vi "Process_donotrun.vi"(8 "error in (no error)":errorcluster, 11 "RemoteControl.ZMQ":refnum<class "RemoteControl.ZMQ.lvclass">) -> (0 "error out":errorcluster, 3 "RemoteControl.ZMQ out":refnum<class "RemoteControl.ZMQ.lvclass">)   [LabVIEW 2019, in "RemoteControl.ZMQ.lvclass"]
doc: "---------------------------------------------------------------\nJKI State Machine Objects™\nhttp://jki.net/state-machine-objects/\nCopyright (C) 2005-2015, JKI <info@jki.net>\nALL RIGHTS RESERVED"
uses:
  RemoteControl.ZMQ.lvclass
  <vilib>/JKI/JKI SMO/SMO/SMO.lvclass
  8787fd3b-6c90-4f4d-93f1-f8fb4481aecc.vi
  <userlib>/LevyLab/RemoteControl/RemoteControl.lvclass
  <userlib>/LevyLab/RemoteControl/Typedefs/Message--Cluster.ctl
  <vilib>/JKI/JKI SMO/SMO/Typedefs/Reserve State--Enum.ctl
  <vilib>/JKI/JKI SMO/SMO/Typedefs/SMOState --Enum.ctl
  <vilib>/JKI/JKI SMO/SMO/Typedefs/Public Events.ctl
  <vilib>/addons/zeromq/zmq_context.lvclass
  <vilib>/addons/zeromq/zmq_socket.lvclass
  <vilib>/addons/zeromq/socket_type.ctl
  <vilib>/addons/zeromq/zeromq.lvlib
  C:/Program Files (x86)/National Instruments/LabVIEW 2019/vi.lib/JKI/JKI SMO/SMO/SMO.lvclass
  C:/Program Files (x86)/National Instruments/LabVIEW 2019/user.lib/LevyLab/RemoteControl/RemoteControl.lvclass
panel:
  in  "endpoint":string="tcp://127.0.0.1:5555"
  out "loop":i32
  in  "stop?":bool
  in  "delay response":bool
  in  "timeout (ms) [500]":i32=500
  out "Message In":string
  in  "stop":bool
  out "Message Out":string
  out "State History":string
  # "remote control"
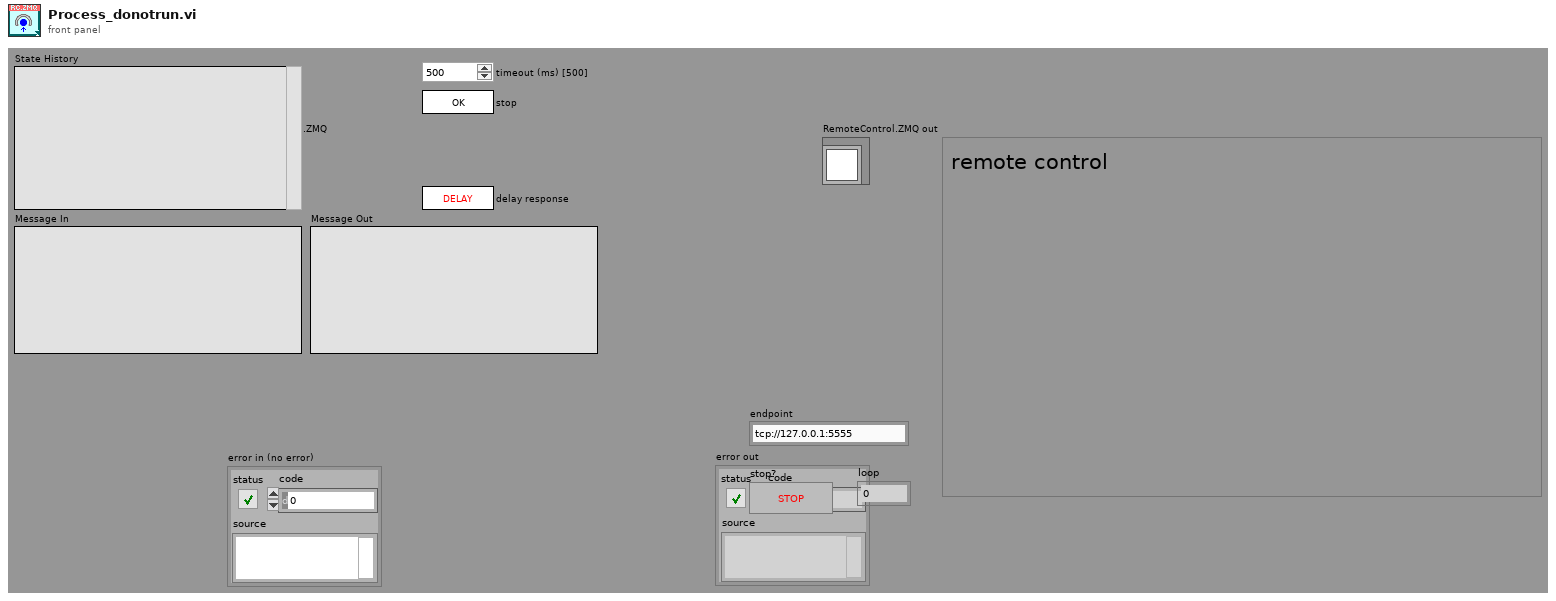
[diagram p1: front panel]
types:
  T1 = enum32{"invalid app kind", "Development System", "Run Time System", "Student Edition", "Embedded LabVIEW", "Evaluation", "Custom"}
  T2 = enum32{"Invalid", "Standard", "Closed", "Hidden", "Minimized", "Maximized"}
  T3 = enum32{"Bad", "Idle", "Run top level", "Running"}
  T4 = typedef "RemoteControl.lvclass/Message--Cluster.ctl" = cluster{"Command":string, "Data":variant, "ID":string}
  T5 = typedef "zeromq.lvlib/socket_type.ctl" = enum8{"ZMQ_PAIR", "ZMQ_PUB", "ZMQ_SUB", "ZMQ_REQ", "ZMQ_REP", "ZMQ_DEALER", "ZMQ_ROUTER", "ZMQ_PULL", "ZMQ_PUSH", "ZMQ_XPUB", "ZMQ_XSUB", "ZMQ_STREAM", "ZMQ_SERVER", "ZMQ_CLIENT", "ZMQ_RADIO", "ZMQ_DISH", "ZMQ_GATHER", "ZMQ_SCATTER", "ZMQ_DGRAM"}
  T6 = cluster{"Core":cluster{"Current VI Reference":refnum<vi>, "Close Panel on Exit?":bool, "Last Error":cluster{"error":errorcluster, "previous state":string, "remaining states":string}, "Shutdown?":bool}, "SelfRef":refnum<class "RemoteControl.ZMQ.lvclass">, "Message (in)":T4, "Message (out)":T4, "state":enum16{"waiting", "processing"}, "to":i32}
  T7 = cluster{"Current VI Reference":refnum<vi>, "Close Panel on Exit?":bool, "Last Error":cluster{"error":errorcluster, "previous state":string, "remaining states":string}, "Shutdown?":bool}
  T8 = typedef "SMO.lvclass/Public Events.ctl" = cluster{"Error":refnum<user-event>, "State":refnum<user-event>, "Reserve State":refnum<user-event>}
  T9 = typedef "SMO.lvclass/Protected Events.ctl" = cluster{"StopProcesses":refnum<user-event>, "AbortProcesses":refnum<user-event>, "Config Changed":refnum<user-event>, "Dependency":refnum<user-event>}
  T10 = typedef "RemoteControl.lvclass/PrivateEvents--Cluster.ctl" = cluster{"Configure":refnum<user-event>, "SendMessageToProcess":refnum<user-event>}
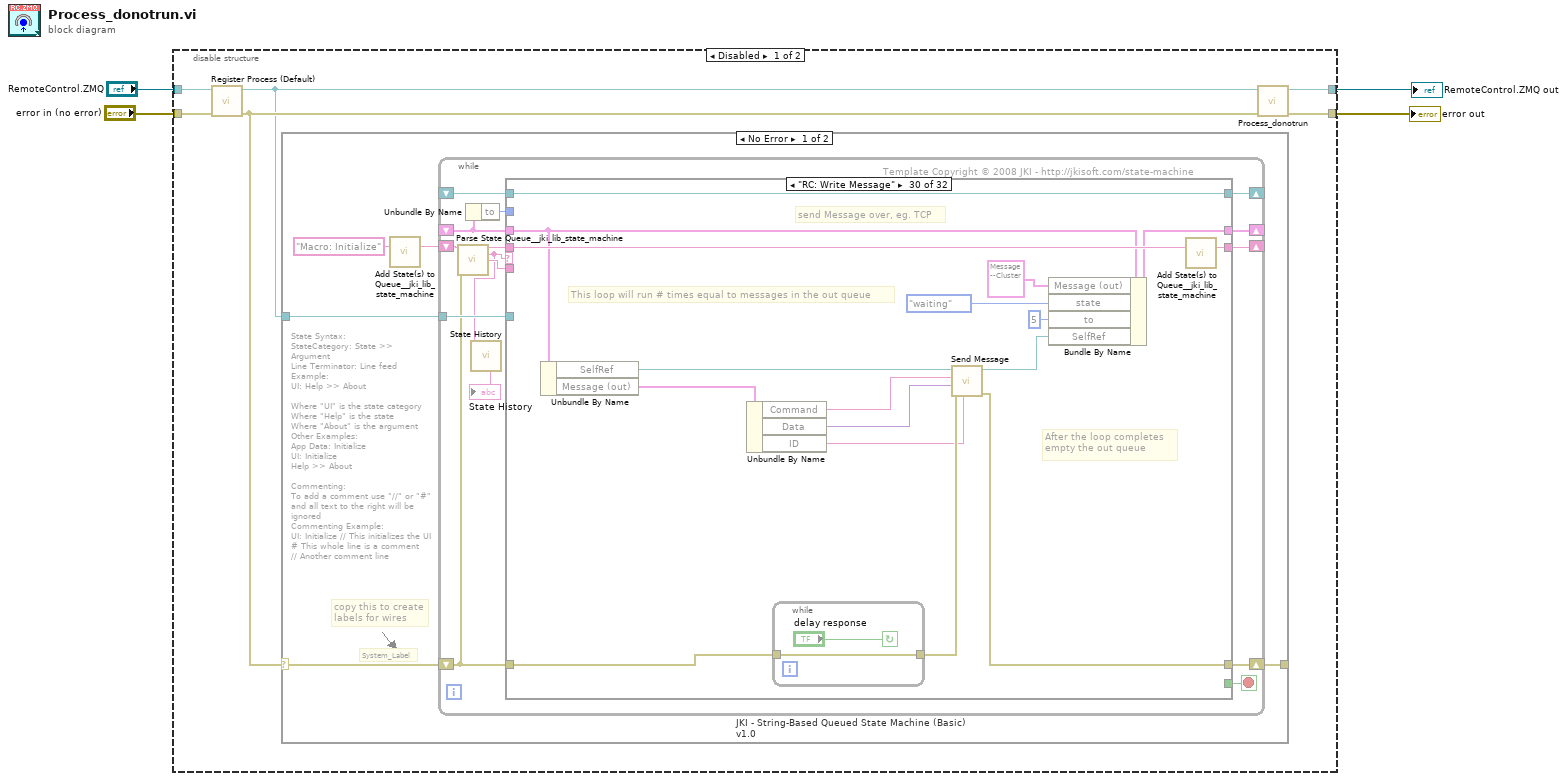
[diagram p0: block diagram]
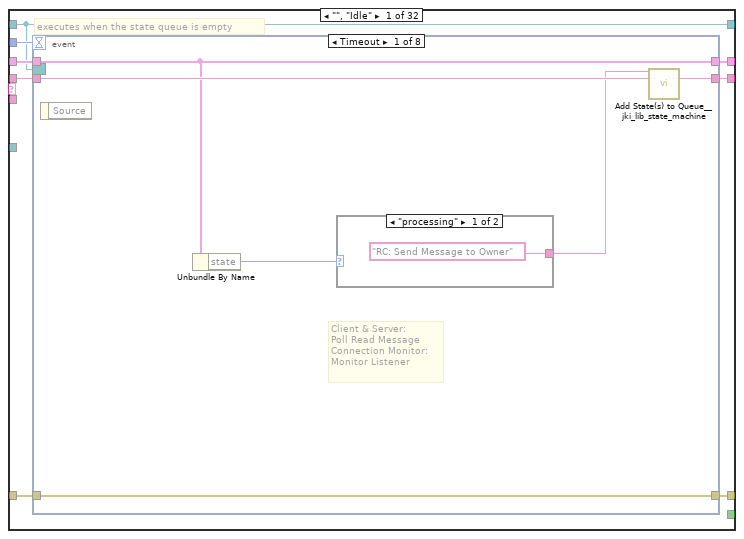
[diagram p2: hidden frame]
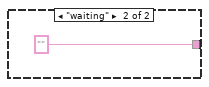
[diagram p3: hidden frame]
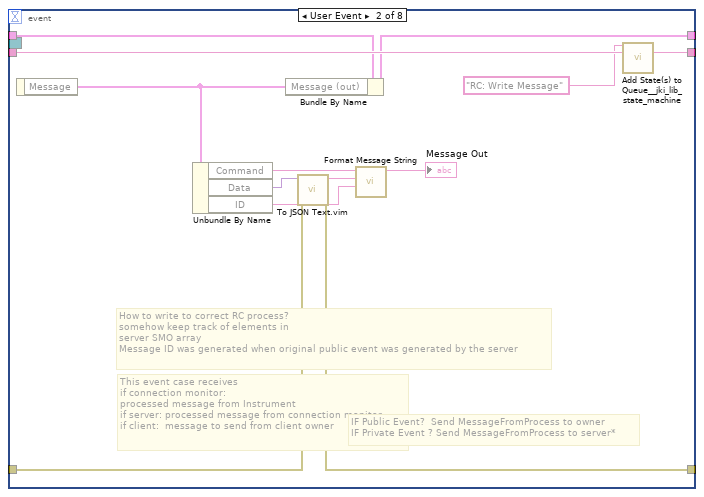
[diagram p4: hidden frame]
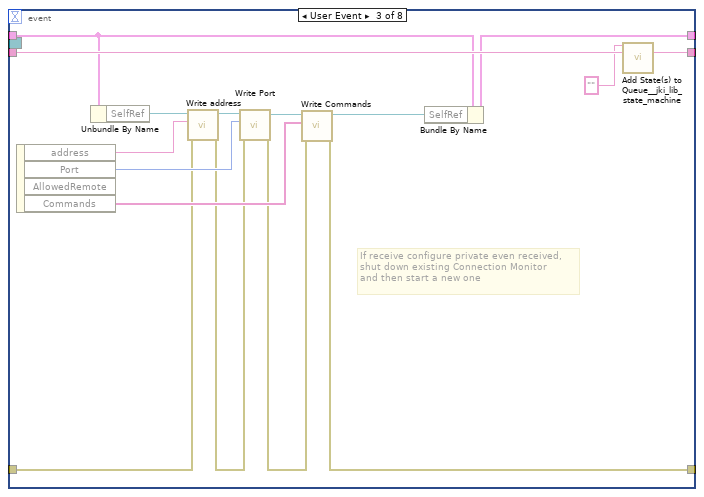
[diagram p5: hidden frame]
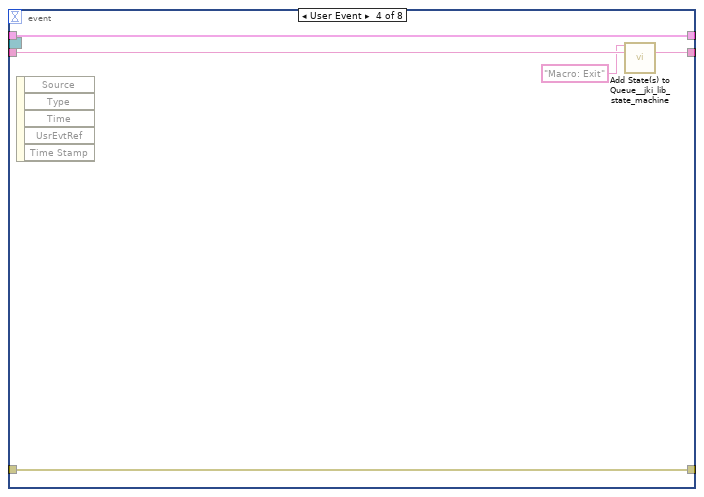
[diagram p6: hidden frame]
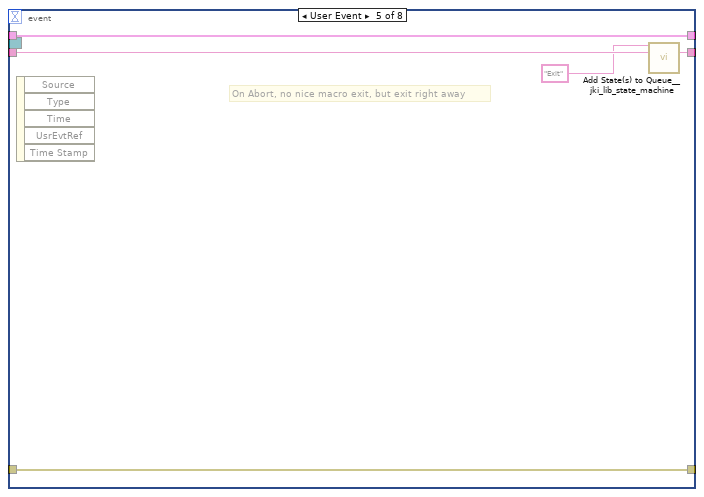
[diagram p7: hidden frame]
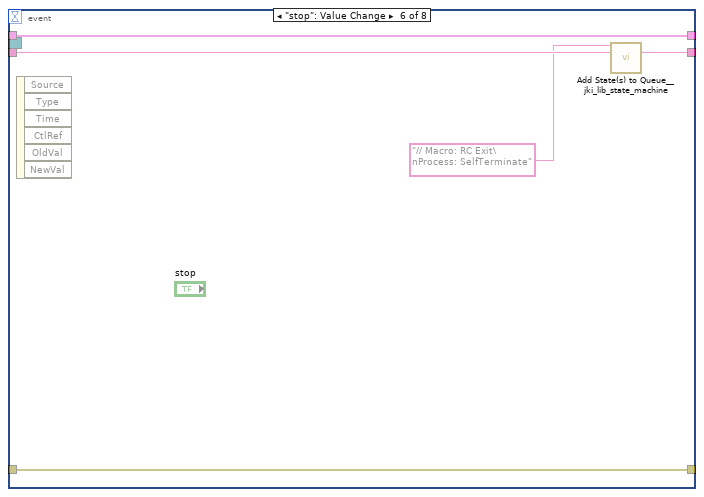
[diagram p8: hidden frame]
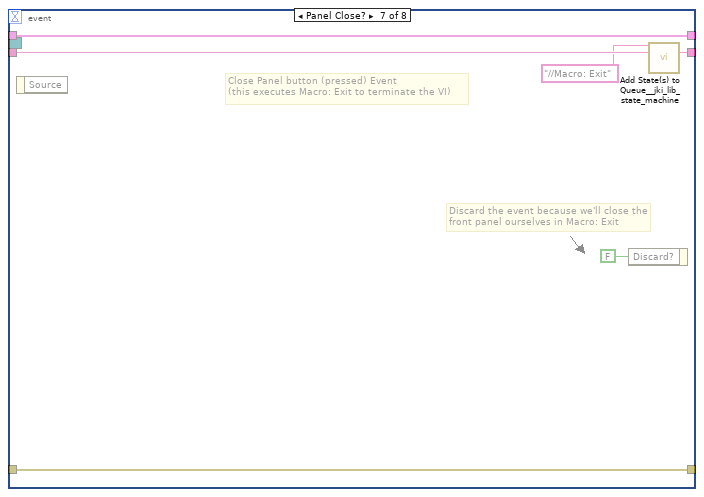
[diagram p9: hidden frame]
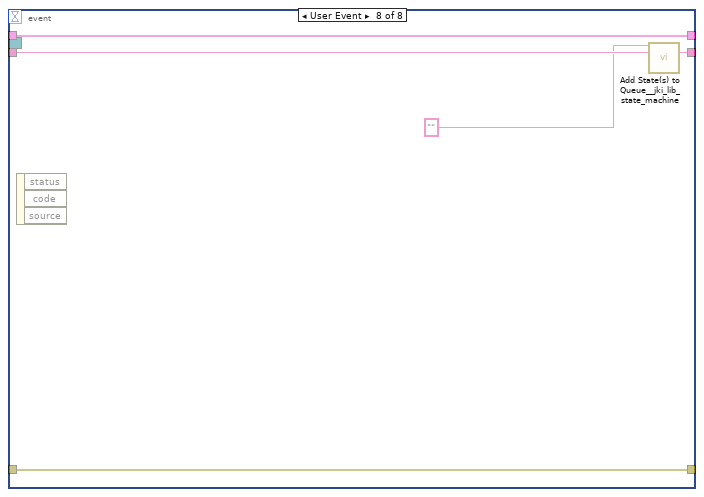
[diagram p10: hidden frame]
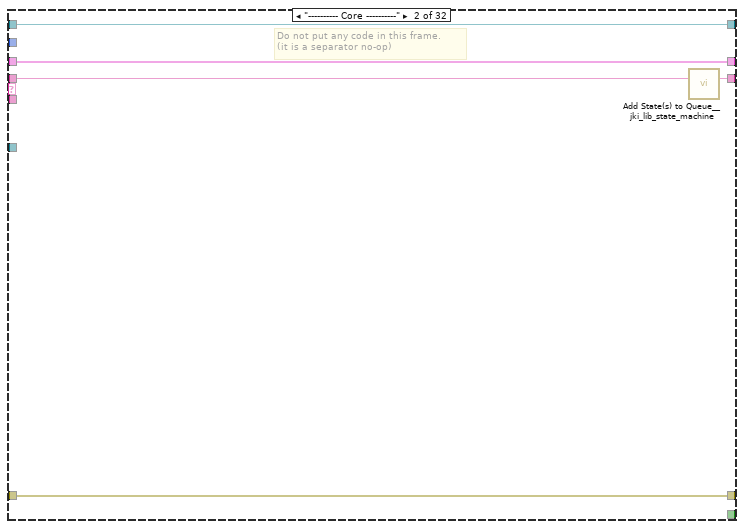
[diagram p11: hidden frame]
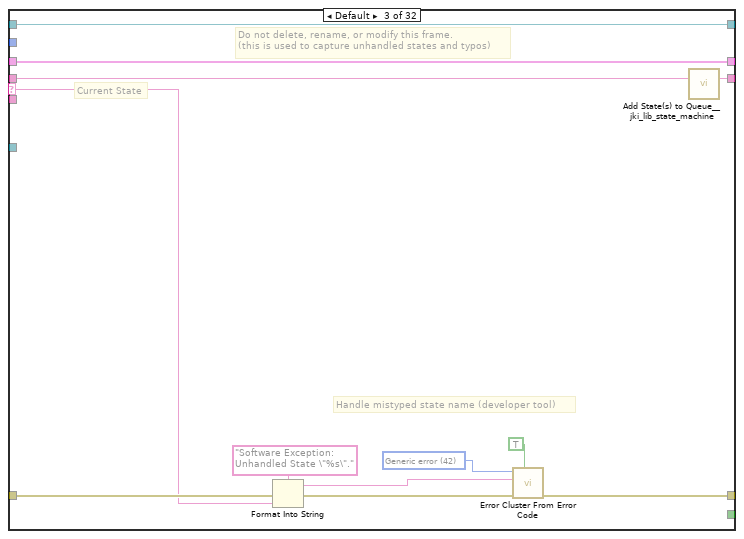
[diagram p12: hidden frame]
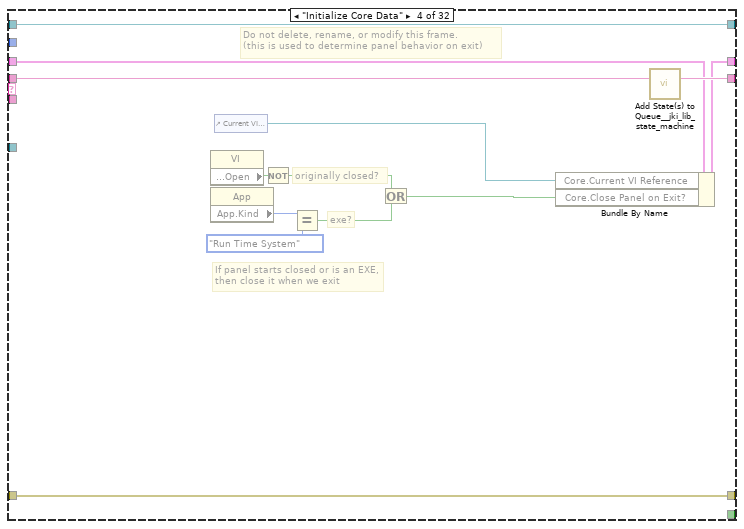
[diagram p13: hidden frame]
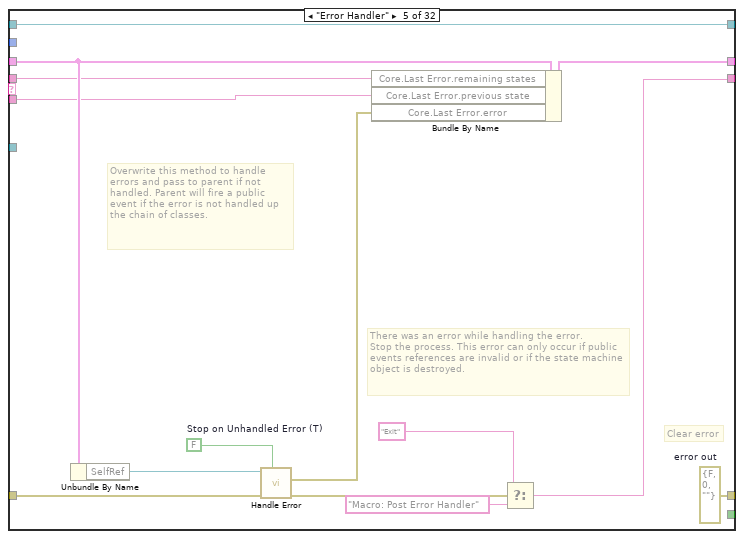
[diagram p14: hidden frame]
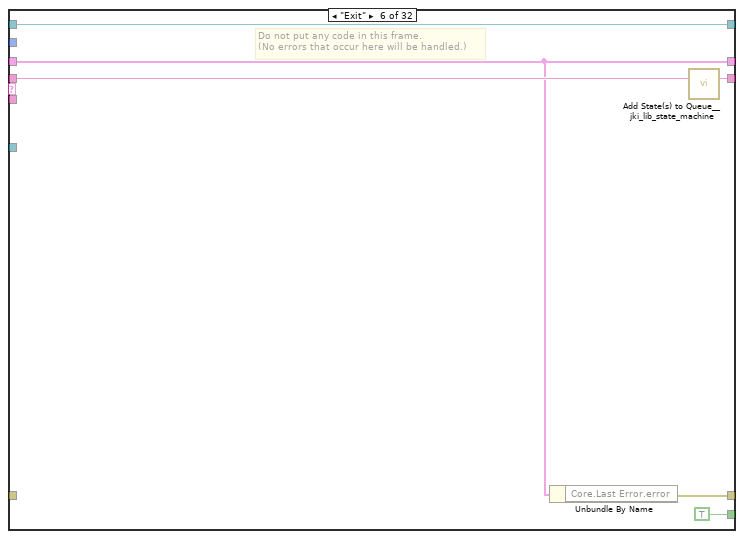
[diagram p15: hidden frame]
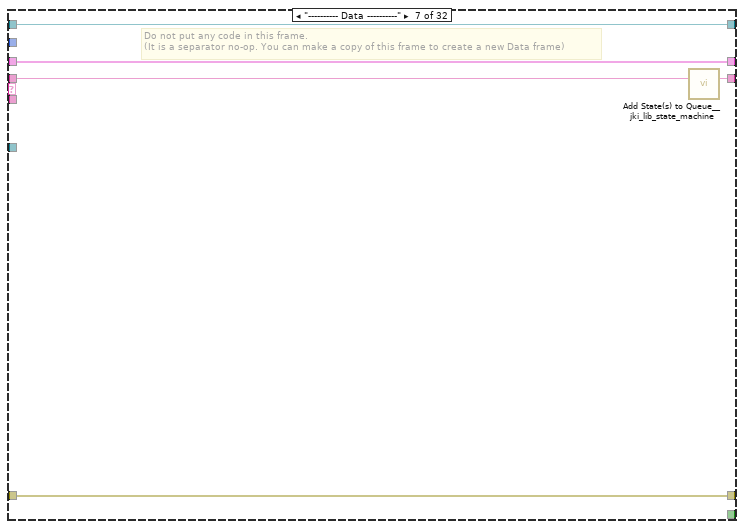
[diagram p16: hidden frame]
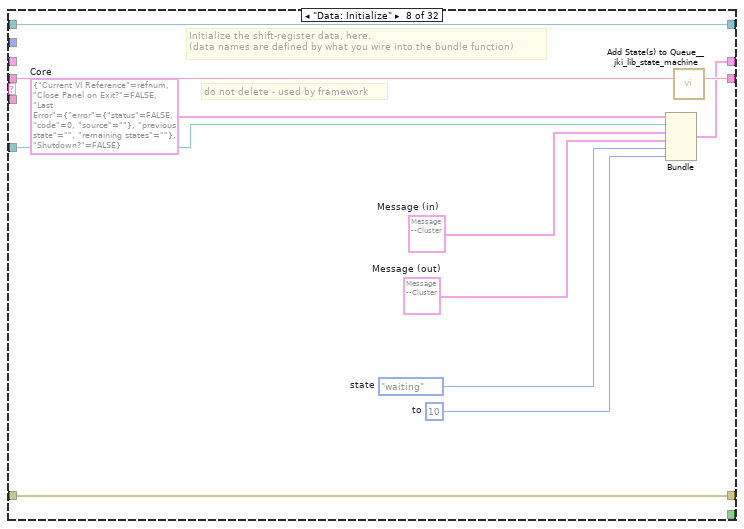
[diagram p17: hidden frame]
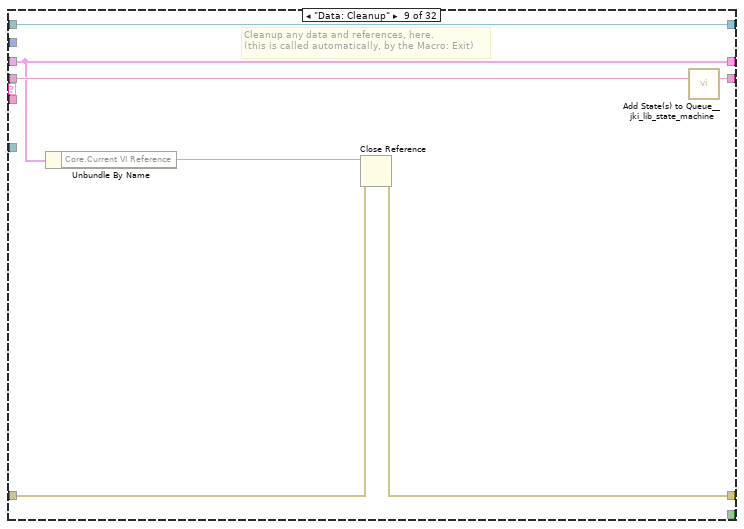
[diagram p18: hidden frame]
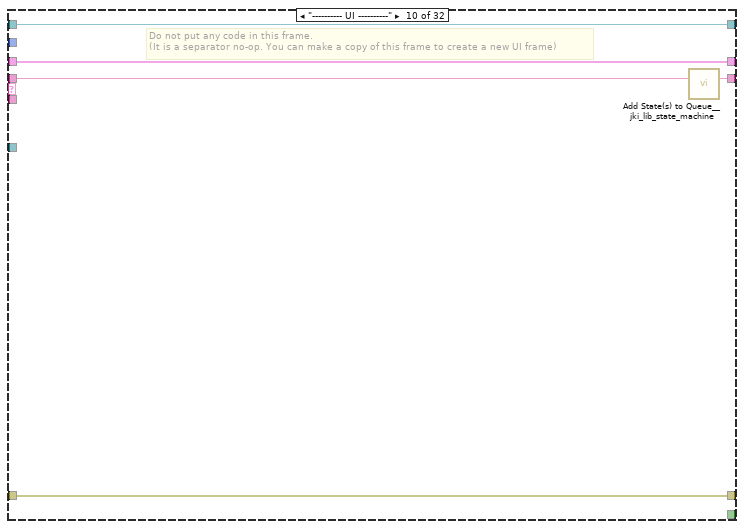
[diagram p19: hidden frame]
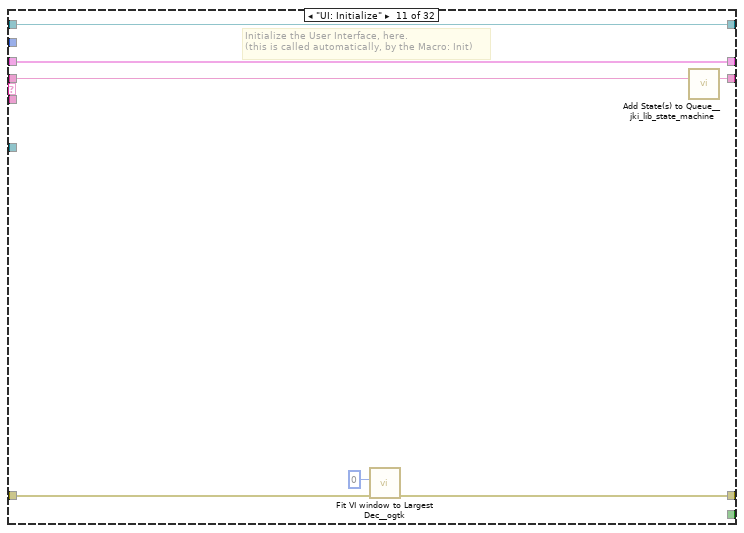
[diagram p20: hidden frame]
diagram:
  n1 = disable-structure shown="Disabled" {
    disable-tunnel: "RemoteControl.ZMQ" -> [w10 w465]
    disable-tunnel: "error in (no error)" -> [w9 w464]
    disable-tunnel: [w6 w465] -> w2
    disable-tunnel: [w5 w464] -> w1
    frame Disabled {
      n2 = call <vilib>:"Register Process (Default).vi"("error in (no error)"=w9, "SMO"=w10) -> ("error out"=w8:errorcluster, "SelfRef"=w7:refnum<class "RemoteControl.ZMQ.lvclass">)  [unwired: 8 in]
      n3 = case shown="No Error" w8 {
        selector: w8 -> [w12 w463]
        tunnel: w7 -> [w13 _]
        tunnel: [w11 w463] -> _
        frame No Error {
          # "State Syntax:\nStateCategory: State >> Argument\nLine Terminator: Line feed\nExample:\nUI: Help >> About\n\nWhere \"UI\" is the state category\nWhere \"Help\" is the state\nWhere \"About\" is the argument\nOther Examples:\nApp Data: Initialize\nUI: Initialize\nHelp >> About\n\nCommenting:\nTo add a comment use \"//\" or \"#\" and all text to the right will be ignored\nCommenting Example:\nUI: Initialize // This initializes the UI\n# This whole line is a comment\n// Another comment line"
          # "copy this to create labels for wires"
          # "System_Label"
          n4 = call <vilib>:"Add State(s) to Queue__jki_lib_state_machine.vi"("State(s) in (\"\")"="Macro: Initialize") -> ("States Out"=w15:string)  [unwired: 14 in]
          n5 = while "JKI - String-Based Queued State Machine (Basic) v1.0" {
            shift-right: [w25] -> _
            shift-left: _ -> [w18]
            shift-right: [w27] -> w11
            shift-left: w12 -> [w21]
            shift-right: [w19] -> _
            shift-left: w15 -> [w28]
            tunnel: w13 -> [w24]
            shift-right: [w23] -> _
            shift-left: _ -> [w22]
            stop <- w26 stop-if-true
            # "Template Copyright © 2008 JKI - http://jkisoft.com/state-machine"
            n6 = call <vilib>:"Parse State Queue__jki_lib_state_machine.vi"("State Queue"=w28, "Error In (no error)"=w21) -> ("Remaining States"=w30:string, "Current State"=w20:string, "Arguments"=w29:string)  [unwired: 11 in]
            n7 = Unbundle By Name(w18) -> ("to"=w17:i32)
            n8 = call <userlib>:"State History.vi"("Current State"=w20) -> ("History"=→"State History":string)  [unwired: 10 in]
            n9 = case shown="\"RC: Write Message\"" w20 {
              selector: w20 -> [_ _ w108 _ _ _ _ _ _ _ _ _ _ _ _ _ _ _ _ _ _ _ _ _ _ _ _ _ _ _ _ _]
              tunnel: w30 -> [w38 w106 w112 w131 w135 w151 w156 w167 w174 w179 w186 w193 w209 w239 w244 w266 w272 w278 w292 w316 w321 w332 w341 w346 w360 w366 w371 w379 w402 w436 w447 w462]
              tunnel: w29 -> [_ _ _ _ w134 _ _ _ _ _ _ w187 w204 _ _ _ _ _ _ _ _ _ _ _ _ _ _ _ _ _ _ _]
              tunnel: [w35 w104 w114 w128 w144 w146 w154 w160 w171 w177 w181 w188 w202 w235 w242 w264 w269 w276 w290 w314 w319 w324 w334 w344 w354 w362 w367 w374 w395 w431 w439 w459] -> w27
              tunnel: [w37 w105 w111 w130 w137 w150 w155 w166 w173 w178 w185 w192 w208 w238 w243 w265 w271 w277 w291 w315 w320 w331 w340 w345 w359 w365 w370 w378 w401 w435 w446 w461] -> w19
              tunnel: [_ _ _ _ _ TRUE _ _ _ _ _ _ _ _ _ _ _ _ _ _ _ _ _ _ _ _ _ _ _ _ _ _] -> w26
              tunnel: [w33 w103 w110 w129 w142 w147 w153 w163 w170 w176 w183 w191 w206 w236 w241 w246 w268 w273 w288 w300 w318 w329 w338 w343 w358 w364 w369 w375 w399 w429 w442 w457] -> w25
              tunnel: w17 -> [w32 _ _ _ _ _ _ _ _ _ _ _ _ _ _ _ _ _ _ _ _ _ _ _ _ _ _ _ _ _ _ _]
              tunnel: w24 -> [_ _ _ _ _ _ _ w157 _ _ _ _ _ _ _ _ _ _ _ _ _ _ _ _ _ _ _ _ _ _ _ _]
              tunnel: [w31 w102 w107 w119 w145 w148 w152 w165 w169 w175 w184 w190 w203 w237 w240 w263 w270 w275 w289 w310 w317 w330 w339 w342 w357 w363 w368 w377 w400 w434 w445 w460] -> w23
              tunnel: w22 -> [w31 w102 w107 w119 w145 w148 w152 w165 w169 w175 w184 w190 w203 w237 w240 w263 w270 w275 w289 w310 w317 w330 w339 w342 _ w363 w368 w377 w400 w434 w445 w460]
              tunnel: w21 -> [w34 w104 w113 w128 w140 _ w154 w160 w172 w177 w180 w189 w207 w235 w242 w264 w269 w276 w290 w314 w319 w325 w335 w344 w355 w362 w367 w373 w385 w432 w440 w449]
              tunnel: w18 -> [w36 w103 w110 w122 w143 w147 w153 _ w170 w176 w183 w191 w206 w236 w241 w246 w268 w273 w286 w299 w318 w329 w333 w343 w358 w364 w369 w375 w387 w430 w443 w456]
              frame "", "Idle" {
                # "executes when the state queue is empty"
                n10 = event shown="[0] Timeout" {
                  selector: w31 -> [_ _ _ _ _ _ _ _]
                  dyn-events: _ -> [_ _ _ _ _ _ _ _]
                  timeout: w32 -> [_ _ _ _ _ _ _ _]
                  tunnel: w38 -> [w44 w59 w75 w80 w85 w89 w96 w101]
                  tunnel: [w43 w58 w74 w79 w84 w90 w95 w100] -> w37
                  tunnel: w36 -> [w40 w55 w66 w77 w82 w88 w93 w98]
                  tunnel: [w42 w48 w60 w78 w83 w86 w94 w99] -> w35
                  tunnel: w34 -> [w42 w47 w62 w78 w83 w86 w94 w99]
                  tunnel: [w40 w57 w73 w77 w82 w88 w93 w98] -> w33
                  event Timeout {
                    # "Client & Server:\nPoll Read Message\nConnection Monitor:\nMonitor Listener"
                    n11 = event-data() -> ()  [unwired: 1 in, 1 out]
                    n12 = Unbundle By Name(w40) -> ("state"=w39:enum16{"waiting", "processing"})
                    n13 = case shown="\"processing\"" w39 {
                      tunnel: ["RC: Send Message to Owner" ("State(s) in Front (\"\")") "" ("State(s) in Front (\"\")")] -> w41
                      frame "processing" {
                      }
                      frame "waiting" {
                      }
                    }
                    n14 = call <vilib>:"Add State(s) to Queue__jki_lib_state_machine.vi"("State(s) in Front (\"\")"=w41, "State(s) in (\"\")"=w44) -> ("States Out"=w43:string)  [unwired: 13 in]
                  }
                  event User Event {
                    # "IF Public Event?  Send MessageFromProcess to owner\nIF Private Event ? Send MessageFromProcess to server*"
                    # "How to write to correct RC process?\nsomehow keep track of elements in\nserver SMO array\nMessage ID was generated when original public event was generated by the server"
                    # "This event case receives\nif connection monitor:\nprocessed message from Instrument\nif server: processed message from connection monitor\nif client:  message to send from client owner"
                    n15 = event-data() -> ("Message"=w49:T4)  [unwired: 1 in]
                    n16 = Unbundle By Name(w49) -> ("Command"=w52:string, "Data"=w51:variant, "ID"=w50:string)
                    n17 = Bundle By Name(cluster=w55, "Message (out)"=w49) -> (w57:T6)
                    n18 = call "To JSON Text.vim"("error in (no error)"=w47, "Anything"=w51) -> ("error out"=w48:errorcluster, "<JSON>"=w53:string)  [unwired: 8 in]
                    n19 = call <userlib>:"Format Message String.vi"("ID"=w50, "Data"=w53, "Command"=w52) -> ("Message"=→"Message Out":string)  [unwired: 8 in]
                    n20 = call <vilib>:"Add State(s) to Queue__jki_lib_state_machine.vi"("State(s) in Front (\"\")"="RC: Write Message" ("State(s) in Front (\"\")"), "State(s) in (\"\")"=w59) -> ("States Out"=w58:string)  [unwired: 13 in]
                  }
                  event User Event {
                    # "If receive configure private even received,\nshut down existing Connection Monitor \nand then start a new one"
                    n21 = event-data() -> ("address"=w64:string, "Port"=w71:u16, "Commands"=w70:string[])  [unwired: 1 in, 1 out]
                    n22 = Unbundle By Name(w66) -> ("SelfRef"=w65:refnum<class "RemoteControl.ZMQ.lvclass">)
                    n23 = call-dynamic "Write address.vi"("error in (no error)"=w62, "address"=w64, "RemoteControl in"=w65) -> ("error out"=w63:errorcluster, "RemoteControl out"=w68:refnum<class "RemoteControl.ZMQ.lvclass">)  [unwired: 7 in]
                    n24 = call-dynamic "Write Port.vi"("error in (no error)"=w63, "Port"=w71, "RemoteControl in"=w68) -> ("error out"=w61:errorcluster, "RemoteControl out"=w69:refnum<class "RemoteControl.ZMQ.lvclass">)  [unwired: 7 in]
                    n25 = call-dynamic "Write Commands.vi"("error in (no error)"=w61, "Commands"=w70, "RemoteControl in"=w69) -> ("error out"=w60:errorcluster, "RemoteControl out"=w67:refnum<class "RemoteControl.ZMQ.lvclass">)  [unwired: 7 in]
                    n26 = Bundle By Name(cluster=w66, "SelfRef"=w67) -> (w73:T6)
                    n27 = call <vilib>:"Add State(s) to Queue__jki_lib_state_machine.vi"("State(s) in Front (\"\")"="" ("State(s) in Front (\"\")"), "State(s) in (\"\")"=w75) -> ("States Out"=w74:string)  [unwired: 13 in]
                  }
                  event User Event {
                    n28 = event-data() -> ()  [unwired: 1 in, 5 out]
                    n29 = call <vilib>:"Add State(s) to Queue__jki_lib_state_machine.vi"("State(s) in Front (\"\")"="Macro: Exit", "State(s) in (\"\")"=w80) -> ("States Out"=w79:string)  [unwired: 13 in]
                  }
                  event User Event {
                    # "On Abort, no nice macro exit, but exit right away"
                    n30 = event-data() -> ()  [unwired: 1 in, 5 out]
                    n31 = call <vilib>:"Add State(s) to Queue__jki_lib_state_machine.vi"("State(s) in Front (\"\")"="Exit", "State(s) in (\"\")"=w85) -> ("States Out"=w84:string)  [unwired: 13 in]
                  }
                  event "stop": Value Change {
                    n32 = event-data() -> ()  [unwired: 1 in, 6 out]
                    n33 = call <vilib>:"Add State(s) to Queue__jki_lib_state_machine.vi"("State(s) in Front (\"\")"="// Macro: RC Exit\nProcess: SelfTerminate" ("State(s) in Front (\"\")"), "State(s) in (\"\")"=w89) -> ("States Out"=w90:string)  [unwired: 13 in]
                  }
                  event Panel Close? {
                    # "Discard the event because we'll close the front panel ourselves in Macro: Exit"
                    # "Close Panel button (pressed) Event\n(this executes Macro: Exit to terminate the VI)"
                    n34 = event-data() -> ()  [unwired: 1 in, 1 out]
                    n35 = event-data("Discard?"=FALSE) -> ()  [unwired: 1 in, 1 out]
                    n36 = call <vilib>:"Add State(s) to Queue__jki_lib_state_machine.vi"("State(s) in Front (\"\")"="//Macro: Exit", "State(s) in (\"\")"=w96) -> ("States Out"=w95:string)  [unwired: 13 in]
                  }
                  event User Event {
                    n37 = event-data() -> ()  [unwired: 1 in, 3 out]
                    n38 = call <vilib>:"Add State(s) to Queue__jki_lib_state_machine.vi"("State(s) in Front (\"\")"="", "State(s) in (\"\")"=w101) -> ("States Out"=w100:string)  [unwired: 13 in]
                  }
                }
              }
              frame "---------- Core ----------" {
                # "Do not put any code in this frame.\n(it is a separator no-op)"
                n39 = call <vilib>:"Add State(s) to Queue__jki_lib_state_machine.vi"("State(s) in (\"\")"=w106) -> ("States Out"=w105:string)  [unwired: 14 in]
              }
              frame Default {
                w117 = 42 items=["No error", "Argument error", "Memory is full", "Out of zone", "End of file", "File already open", "Generic file I/O error", "File not found", "File permission error", "Disk is full", "Duplicate path", "Too many files open", "System feature not enabled", "Resource file not found", "Cannot add resource", "Resource not found", "Image not found", "Image memory error", "Pen does not exist", "Config type invalid", "Config token not found", "Config parse error", "Config memory error", "Bad external code format", "Bad external code offset", "External code not present", "Null window", "Destroy window error", "Null menu", "Print aborted", "Bad print record", "Print driver error", "Windows error during printing", "Memory error during printing", "Print dialog error", "Generic print error", "Invalid device refnum", "Device not found", "Device parameter error", "Device unit error", "Cannot open device", "Device call aborted", "Generic error", "Cancelled by user", "Object ID too low", "Object ID too high", "Object not in heap", "Unknown heap", "Unknown object (invalid DefProc)", "Unknown object (DefProc not in table)", "Message out of range", "Invalid (null) method", "Unknown message", "Manager call not supported", "Bad address", "Network operation in progress", "Network operation timed out", "Connection is busy", "Network attribute not supported", "Network error", "Address in use", "System out of memory", "Connection aborted", "Connection refused", "Not connected", "Already connected", "Connection closed", "Initialization error (interapplication manager)", "Bad occurrence", "Wait on unbound occurrence handler", "Occurrence queue overflow", "Datalog type conflict", "Unused", "Unrecognized type (interapplication manager)", "Memory corrupt", "Failed to make temporary DLL", "Old CIN version", "Drag socket not found", "Failed to load drop-object", "Failed to register OLE object", "Failed to release OLE object", "Format specifier type mismatch", "Unknown format specifier", "Too few format specifiers", "Too many format specifiers", "Scan failed", "Newer CIN version", "Error converting to variant", "Runtime menu error", "Password tampered", "Variant attribute not found", "Incompatible variant data type", "Event data is not available", "Event Store is not present", "Occurrence is not found", "Event Queue is not created", "Event info is not available", "Refnum passed is NULL", "Error retrieving Class GUID", "Error retrieving CoClass GUID", "Error retrieving TypeLib GUID.", "Bad built application magic bytes.", "Specific driver is different from the specific driver associated with the Logical Name.", "There is no session opened to the class driver.", "Max Error", "MAX - Error with config objects", "MAX - Error loading configuration", "MAX - Group not supported"]
                # "Current State"
                # "Do not delete, rename, or modify this frame.\n(this is used to capture unhandled states and typos)"
                # "Handle mistyped state name (developer tool)"
                n40 = Format Into String(format string="Software Exception: Unhandled State \"%s\"." ("message"), error in=w113, w108) -> (resulting string=w116:string, error out=w115:errorcluster)  [unwired: 1 in]
                n41 = call <vilib>:"Error Cluster From Error Code.vi"("show call chain? (False)"=TRUE, "error in (no error)"=w115, "error message (\"\")"=w116, "error code (0)"=w117) -> ("error out"=w114:errorcluster)  [unwired: 5 in]
                n42 = call <vilib>:"Add State(s) to Queue__jki_lib_state_machine.vi"("State(s) in (\"\")"=w112) -> ("States Out"=w111:string)  [unwired: 14 in]
              }
              frame "Initialize Core Data" {
                # "Do not delete, rename, or modify this frame.\n(this is used to determine panel behavior on exit)"
                # "originally closed?"
                # "exe?"
                # "If panel starts closed or is an EXE, then close it when we exit"
                n43 = property class="VI"() -> ("Front Panel.Open"=w127:bool)  [unwired: 2 in, 2 out]
                n44 = property class="App"() -> ("App.Kind"=w126:T1)  [unwired: 2 in, 2 out]
                n45 = control-ref of="Current VI Reference"() -> (w120:refnum<vi>)
                n46 = Not(x=w127) -> (.not. x?=w124:bool)
                n47 = Equal?(x=w126, y=T1."Run Time System" ("Application:Kind")) -> (x = y?=w123:bool)
                n48 = Or(x=w124, y=w123) -> (x .or. y?=w121:bool)
                n49 = Bundle By Name(cluster=w122, "Core.Current VI Reference"=w120, "Core.Close Panel on Exit?"=w121) -> (w129:T6)
                n50 = call <vilib>:"Add State(s) to Queue__jki_lib_state_machine.vi"("State(s) in (\"\")"=w131) -> ("States Out"=w130:string)  [unwired: 14 in]
              }
              frame "Error Handler" {
                w141 = FALSE  # Stop on Unhandled Error (T)
                w144 = errorcluster {"status"=FALSE, "code"=0, "source"=""}  # error out
                # "There was an error while handling the error.\nStop the process. This error can only occur if public events references are invalid or if the state machine object is destroyed."
                # "Clear error"
                # "Overwrite this method to handle errors and pass to parent if not handled. Parent will fire a public event if the error is not handled up the chain of classes."
                n51 = Unbundle By Name(w143) -> ("SelfRef"=w139:refnum<class "RemoteControl.ZMQ.lvclass">)
                n52 = call-dynamic "Handle Error.vi"("Stop on Unhandled Error (T)"=w141, "error in"=w140, "SMO"=w139) -> ("handling error"=w132:errorcluster, "Unhandled error"=w133:errorcluster)  [unwired: 6 in, 1 out]
                n53 = Bundle By Name(cluster=w143, "Core.Last Error.remaining states"=w135, "Core.Last Error.previous state"=w134, "Core.Last Error.error"=w133) -> (w142:T6)
                n54 = Select(t="Exit", s=w132, f="Macro: Post Error Handler") -> (s? t:f=w137:string)
              }
              frame "Exit" {
                # "Do not put any code in this frame.\n(No errors that occur here will be handled.)"
                n55 = Unbundle By Name(w147) -> ("Core.Last Error.error"=w146:errorcluster)
                n56 = call <vilib>:"Add State(s) to Queue__jki_lib_state_machine.vi"("State(s) in (\"\")"=w151) -> ("States Out"=w150:string)  [unwired: 14 in]
              }
              frame "---------- Data ----------" {
                # "Do not put any code in this frame.\n(It is a separator no-op. You can make a copy of this frame to create a new Data frame)"
                n57 = call <vilib>:"Add State(s) to Queue__jki_lib_state_machine.vi"("State(s) in (\"\")"=w156) -> ("States Out"=w155:string)  [unwired: 14 in]
              }
              frame "Data: Initialize" {
                w158 = 10  # to
                w159 = enum16{"waiting", "processing"}."waiting"  # state
                w161 = T4 {"Command"="", "Data"=variant, "ID"=""}  # Message (out)
                w162 = T4 {"Command"="", "Data"=variant, "ID"=""}  # Message (in)
                w164 = T7 {"Current VI Reference"=refnum, "Close Panel on Exit?"=FALSE, "Last Error"={"error"={"status"=FALSE, "code"=0, "source"=""}, "previous state"="", "remaining states"=""}, "Shutdown?"=FALSE}  # Core
                # "do not delete - used by framework"
                # "Initialize the shift-register data, here.\n(data names are defined by what you wire into the bundle function)"
                n58 = Bundle("Core"=w164, "SelfRef"=w157, "Message (in)"=w162, "Message (out)"=w161, "state"=w159, "to"=w158) -> (w163:T6)  [unwired: 1 in]
                n59 = call <vilib>:"Add State(s) to Queue__jki_lib_state_machine.vi"("State(s) in (\"\")"=w167) -> ("States Out"=w166:string)  [unwired: 14 in]
              }
              frame "Data: Cleanup" {
                # "Cleanup any data and references, here.\n(this is called automatically, by the Macro: Exit)"
                n60 = Unbundle By Name(w170) -> ("Core.Current VI Reference"=w168:refnum<vi>)
                n61 = Close Reference(reference=w168, error in (no error)=w172) -> (error out=w171:errorcluster)
                n62 = call <vilib>:"Add State(s) to Queue__jki_lib_state_machine.vi"("State(s) in (\"\")"=w174) -> ("States Out"=w173:string)  [unwired: 14 in]
              }
              frame "---------- UI ----------" {
                # "Do not put any code in this frame.\n(It is a separator no-op. You can make a copy of this frame to create a new UI frame)"
                n63 = call <vilib>:"Add State(s) to Queue__jki_lib_state_machine.vi"("State(s) in (\"\")"=w179) -> ("States Out"=w178:string)  [unwired: 14 in]
              }
              frame "UI: Initialize" {
                # "Initialize the User Interface, here.\n(this is called automatically, by the Macro: Init)"
                n64 = call <userlib>:"Fit VI window to Largest Dec__ogtk.vi"("error in (no error)"=w180, "border spacing (2 px)"=0) -> ("error out"=w181:errorcluster)  [unwired: 4 in, 1 out]
                n65 = call <vilib>:"Add State(s) to Queue__jki_lib_state_machine.vi"("State(s) in (\"\")"=w186) -> ("States Out"=w185:string)  [unwired: 14 in]
              }
              frame "UI: Cursor Set" {
                # "Argument"
                # "Initialize the User Interface, here.\n(this is called automatically, by the Macro: Init)"
                n66 = disable-structure shown="Default" {
                  disable-tunnel: w189 -> [w194 w197]
                  disable-tunnel: [w194 w196] -> w188
                  disable-tunnel: w187 -> [_ w195]
                  frame condition #0 {
                  }
                  frame condition #1 (active) {
                    n67 = case shown="\"Idle\", Default" w195 {
                      tunnel: w197 -> [w199 w201]
                      tunnel: [w198 w200] -> w196
                      frame "Idle", Default {
                        n68 = call <vilib>:"Unset Busy.vi"("error in (no error)"=w199) -> ("error out"=w198:errorcluster)  [unwired: 10 in]
                      }
                      frame "Busy" {
                        n69 = call <vilib>:"Set Busy.vi"("error in (no error)"=w201) -> ("error out"=w200:errorcluster)  [unwired: 9 in, 1 out]
                      }
                    }
                  }
                }
                n70 = call <vilib>:"Add State(s) to Queue__jki_lib_state_machine.vi"("State(s) in (\"\")"=w193) -> ("States Out"=w192:string)  [unwired: 14 in]
              }
              frame "UI: Front Panel State" {
                # "Argument"
                # "Set Front Panel Open or Closed\n(Usage: \"UI: Front Panel State >> Open|Close\")"
                n71 = Unbundle By Name(w206) -> ("Core.Current VI Reference"=w205:refnum<vi>)
                n72 = disable-structure shown="Default" {
                  disable-tunnel: w207 -> [w213 w234]
                  disable-tunnel: [w212 w234] -> w202
                  disable-tunnel: w205 -> [w211 _]
                  disable-tunnel: w204 -> [w210 _]
                  frame condition #0 (active) {
                    n73 = case shown="\"Close\"" w210 {
                      tunnel: w213 -> [w217 w228]
                      tunnel: [w218 w229] -> w212
                      tunnel: w211 -> [_ _]
                      frame "Open", Default {
                        n74 = property class="VI"(error in=w217) -> (reference out=w215:refnum<vi>, error out=w216:errorcluster, "FP.State"=w214:T2)  [unwired: 1 in]
                        n75 = case shown="\"Closed\"" w214 {
                          tunnel: [w221 w224] -> w218
                          tunnel: w216 -> [w220 w224]
                          tunnel: w215 -> [w219 _]
                          frame "Closed" {
                            n76 = invoke class="VI" method="FP.Open"(reference=w219, error in=w220, "Activate"=TRUE, "State"=T2."Standard") -> (error out=w221:errorcluster)  [unwired: 1 in, 4 out]
                          }
                          frame Default {
                          }
                        }
                      }
                      frame "Close" {
                        n77 = property class="VI"(error in=w228) -> (reference out=w226:refnum<vi>, error out=w227:errorcluster, "FP.State"=w225:T2)  [unwired: 1 in]
                        n78 = case shown="Default" w225 {
                          tunnel: [w230 w233] -> w229
                          tunnel: w227 -> [w230 w232]
                          tunnel: w226 -> [_ w231]
                          frame "Invalid", "Closed" {
                          }
                          frame Default {
                            n79 = invoke class="VI" method="FP.Close"(reference=w231, error in=w232) -> (error out=w233:errorcluster)  [unwired: 1 in, 2 out]
                          }
                        }
                      }
                    }
                  }
                  frame condition #1 {
                  }
                }
                n80 = call <vilib>:"Add State(s) to Queue__jki_lib_state_machine.vi"("State(s) in (\"\")"=w209) -> ("States Out"=w208:string)  [unwired: 14 in]
              }
              frame "UI: Wait" {
                # "Do not put any code in this frame.\n(It is a separator no-op. You can make a copy of this frame to create a new UI frame)"
                n81 = call <vilib>:"Add State(s) to Queue__jki_lib_state_machine.vi"("State(s) in (\"\")"=w239) -> ("States Out"=w238:string)  [unwired: 14 in]
              }
              frame "---------- Macro ----------" {
                # "Do not put any code in this frame.\n(It is a separator no-op. You can make a copy of this frame to create a new Macro frame)"
                n82 = call <vilib>:"Add State(s) to Queue__jki_lib_state_machine.vi"("State(s) in (\"\")"=w244) -> ("States Out"=w243:string)  [unwired: 14 in]
              }
              frame "Macro: Initialize" {
                w255 = "Process: Sync"
                # "This needs to be called before Data: Initialize"
                # "Initialization Macro\n(This is called once, when the VI starts)"
                n83 = control-ref of="This VI"() -> (w257:refnum<vi>)
                n84 = property class="VI"(reference=w257) -> ("Exec.State"=w256:T3)  [unwired: 1 in, 2 out]
                n85 = Equal?(x=w256, y=T3."Run top level") -> (x = y?=w261:bool)
                n86 = Select(t="Open", s=TRUE, f="Close") -> (s? t:f=w252:string)
                n87 = Select(t=w255, s=w261, f="") -> ()  [unwired: 1 out]
                n88 = call <vilib>:"Build State String with Arguments__JKI_lib_State_Machine.vi"("Arguments (\"\")"=w252, "State"="UI: Front Panel State") -> ("State with Arguments"=w249:string)  [unwired: 4 in]
                n89 = call <vilib>:"Add State(s) to Queue__jki_lib_state_machine.vi"("State(s) in Front (\"\")"="UI: Initialize", "State(s) in (\"\")"=w249, "State(s) at Back (\"\")"="UI: Wait\nMacro: RC Initialize") -> ("States Out"=w247:string)  [unwired: 12 in]
                n90 = call <vilib>:"Add State(s) to Queue__jki_lib_state_machine.vi"("State(s) in Front (\"\")"="Data: Initialize\nInitialize Core Data\nEvents: Register", "State(s) in (\"\")"=w255, "State(s) at Back (\"\")"=w247) -> ("States Out"=w258:string)  [unwired: 12 in]
                n91 = call <vilib>:"Add State(s) to Queue__jki_lib_state_machine.vi"("State(s) in Front (\"\")"=w258, "State(s) in (\"\")"=w266) -> ("States Out"=w265:string)  [unwired: 13 in]
              }
              frame "Macro: RC Initialize" {
                n92 = call <vilib>:"Add State(s) to Queue__jki_lib_state_machine.vi"("State(s) in Front (\"\")"="RC: Open Server Connection" ("State(s) in Front (\"\")"), "State(s) in (\"\")"=w272) -> ("States Out"=w271:string)  [unwired: 13 in]
              }
              frame "Macro: RC Exit" {
                n93 = call <vilib>:"Add State(s) to Queue__jki_lib_state_machine.vi"("State(s) in Front (\"\")"="RC: Close Connection" ("State(s) in Front (\"\")"), "State(s) in (\"\")"=w278) -> ("States Out"=w277:string)  [unwired: 13 in]
              }
              frame "Macro: Post Error Handler" {
                # "Clear Last Error?"
                n94 = Unbundle By Name(w286) -> ("Core.Last Error.error"=w282:errorcluster)
                n95 = Unbundle By Name(w286) -> ("Core.Last Error.remaining states"=w285:string, "Core.Shutdown?"=w284:bool)
                n96 = case shown="False" FALSE {
                  tunnel: w282 -> [w293 _]
                  tunnel: [w293 _] -> w280
                  frame False {
                  }
                  frame True {
                  }
                }
                n97 = case shown="True" w284 {
                  tunnel: w285 -> [_ w296]
                  tunnel: ["Macro: RC Exit\nMacro: RC Initialize" ("State(s) in Front (\"\")") w295] -> w283
                  frame False {
                    # "These are the remaining states (at the moment the error occured). States can be altered according to business logic."
                    # "NOT SHUTTING DOWN"
                  }
                  frame True {
                    # "Developer can decide to alter the states but should be aware that during the shutdown process, there are certain states that must be run for the SMO to properly shut itself (and this process) down. As such, one can add states to perform additional clean-ups, but should append the remaining state to be executed."
                    # "SHUTTING DOWN"
                    n98 = call <vilib>:"Add State(s) to Queue__jki_lib_state_machine.vi"("State(s) in (\"\")"=w296) -> ("States Out"=w295:string)  [unwired: 14 in]
                  }
                }
                n99 = Bundle By Name(cluster=w286, "Core.Last Error.error"=w280, "Message (out)"=T4 {"Command"="", "Data"=variant, "ID"=""} ("Messages (out)"), "state"=enum16{"waiting", "processing"}."waiting") -> (w288:T6)
                n100 = call <vilib>:"Add State(s) to Queue__jki_lib_state_machine.vi"("State(s) in Front (\"\")"=w283, "State(s) in (\"\")"=w292) -> ("States Out"=w291:string)  [unwired: 13 in]
              }
              frame "Macro: Exit" {
                # "Exit Macro\n(This is called once, when the VI exits)"
                n101 = Unbundle By Name(w299) -> ("Core.Close Panel on Exit?"=w306:bool)
                n102 = Select(t="Open", s=TRUE, f="Close") -> (s? t:f=w303:string)
                n103 = call <vilib>:"Build State String with Arguments__JKI_lib_State_Machine.vi"("Arguments (\"\")"=w303, "State"="UI: Front Panel State") -> ("State with Arguments"=w301:string)  [unwired: 4 in]
                n104 = Bundle By Name(cluster=w299, "Core.Shutdown?"=TRUE) -> (w300:T6)
                n105 = Select(t=w301, s=w306, f="") -> (s? t:f=w312:string)
                n106 = call <vilib>:"Add State(s) to Queue__jki_lib_state_machine.vi"("State(s) in Front (\"\")"="Macro: RC Exit", "State(s) at Back (\"\")"="Data: Cleanup\nEvents: Unregister\nProcess: Sync\nExit") -> ("States Out"=w307:string)  [unwired: 13 in]
                n107 = call <vilib>:"Add State(s) to Queue__jki_lib_state_machine.vi"("State(s) in (\"\")"=w312, "State(s) at Back (\"\")"=w307) -> ("States Out"=w311:string)  [unwired: 13 in]
                n108 = call <vilib>:"Add State(s) to Queue__jki_lib_state_machine.vi"("State(s) in Front (\"\")"=w311, "State(s) in (\"\")"=w316) -> ("States Out"=w315:string)  [unwired: 13 in]
              }
              frame "---------- Process ----------" {
                # "Template Separator\n(You can make a copy of, or modify, this frame)"
                n109 = call <vilib>:"Add State(s) to Queue__jki_lib_state_machine.vi"("State(s) in (\"\")"=w321) -> ("States Out"=w320:string)  [unwired: 14 in]
              }
              frame "Process: Sync" {
                n110 = Unbundle By Name(w329) -> ("SelfRef"=w322:refnum<class "RemoteControl.ZMQ.lvclass">)
                n111 = call <vilib>:"WaitOnProcessSync.vi"("error in (no error)"=w325, "SMO"=w322) -> ("error out"=w324:errorcluster, "Don't run?"=w328:bool)  [unwired: 7 in, 1 out]
                n112 = Select(t="Data: Cleanup\nEvents: Unregister\nExit", s=w328, f="") -> (s? t:f=w323:string)
                n113 = call <vilib>:"Add State(s) to Queue__jki_lib_state_machine.vi"("State(s) in Front (\"\")"=w323, "State(s) in (\"\")"=w332) -> ("States Out"=w331:string)  [unwired: 13 in]
              }
              frame "Process: SelfTerminate" {
                n114 = Unbundle By Name(w333) -> ("SelfRef"=w337:refnum<class "RemoteControl.ZMQ.lvclass">)
                n115 = call <vilib>:"SelfTerminate.vi"("error in (no error)"=w335, "SMO in"=w337) -> ("error out"=w334:errorcluster, "SMO out"=w336:refnum<class "RemoteControl.ZMQ.lvclass">)  [unwired: 8 in]
                n116 = Bundle By Name(cluster=w333, "SelfRef"=w336) -> (w338:T6)
                n117 = call <vilib>:"Add State(s) to Queue__jki_lib_state_machine.vi"("State(s) in (\"\")"=w341) -> ("States Out"=w340:string)  [unwired: 14 in]
              }
              frame "---------- Events ----------" {
                # "Template Separator\n(You can make a copy of, or modify, this frame)"
                n118 = call <vilib>:"Add State(s) to Queue__jki_lib_state_machine.vi"("State(s) in (\"\")"=w346) -> ("States Out"=w345:string)  [unwired: 14 in]
              }
              frame "Events: Register" {
                w348 = T8 {"Error"=refnum, "State"=refnum, "Reserve State"=refnum}  # Listener Public Events
                # "Expand to add\nmore events"
                n119 = Unbundle By Name(w358) -> ("SelfRef"=w347:refnum<class "RemoteControl.ZMQ.lvclass">)
                n120 = call <vilib>:"GetProtectedEvents.vi"("SMO"=w347) -> ("error out"=w352:errorcluster, "SMO Protected Events"=w356:T9, "SMO out"=w350:refnum<class "RemoteControl.ZMQ.lvclass">)  [unwired: 8 in]
                n121 = call <userlib>:"RemoteControl.GetPrivateEvents.vi"("RemoteControl"=w350) -> ("error out"=w351:errorcluster, "RC Private Events"=w349:T10)  [unwired: 8 in, 1 out]
                n122 = register-events(w356, w349, w348) -> (reference out=w357:refnum<event-registration>, error out=w353:errorcluster)  [unwired: 2 in]
                n123 = Merge Errors(w351, w355, w353, w352) -> (w354:errorcluster)
                n124 = call <vilib>:"Add State(s) to Queue__jki_lib_state_machine.vi"("State(s) in (\"\")"=w360) -> ("States Out"=w359:string)  [unwired: 14 in]
              }
              frame "Events: Unregister" {
                n125 = Unregister For Events(event registration refnum=w363, error in=w362) -> (error out=w361:errorcluster)
                n126 = call <vilib>:"Clear Errors.vi"("error in (no error)"=w361) -> ()  [unwired: 5 in, 2 out]
                n127 = call <vilib>:"Add State(s) to Queue__jki_lib_state_machine.vi"("State(s) in (\"\")"=w366) -> ("States Out"=w365:string)  [unwired: 14 in]
              }
              frame "---------- RC ----------" {
                # "Template Separator\n(You can make a copy of, or modify, this frame)"
                n128 = call <vilib>:"Add State(s) to Queue__jki_lib_state_machine.vi"("State(s) in (\"\")"=w371) -> ("States Out"=w370:string)  [unwired: 14 in]
              }
              frame "RC: Send Message to Owner" {
                # "Send Message to Owner to be processed\n(Send a message to the instrument to be processed)"
                n129 = Unbundle By Name(w375) -> ("SelfRef"=w376:refnum<class "RemoteControl.ZMQ.lvclass">, "Message (in)"=w372:T4)
                n130 = call <userlib>:"RemoteControl.SendMessageFromProcess.vi"("error in (no error)"=w373, "Message"=w372, "RemoteControl"=w376) -> ("error out"=w374:errorcluster)  [unwired: 7 in, 1 out]
                n131 = call <vilib>:"Add State(s) to Queue__jki_lib_state_machine.vi"("State(s) in (\"\")"=w379) -> ("States Out"=w378:string)  [unwired: 14 in]
              }
              frame "RC: Read Message" {
                # "poll the number\nof open connections"
                # "Read Message over, eg TCP"
                # "If command is empty do not Send Message"
                n132 = Unbundle By Name(w387) -> ("SelfRef"=w386:refnum<class "RemoteControl.ZMQ.lvclass">)
                n133 = Unbundle By Name(w387) -> ("to"=w393:i32)
                n134 = call <userlib>:"Write Timeout.vi"("error in (no error)"=w385, "timeout (ms) [500]"="timeout (ms) [500]", "RemoteControl in"=w386) -> ("error out"=w384:errorcluster, "RemoteControl out"=w383:refnum<class "RemoteControl.ZMQ.lvclass">)  [unwired: 7 in]
                n135 = call-dynamic "Read Message.vi"("error in (no error)"=w384, "RemoteControl.ZMQ in"=w383) -> ("error out"=w391:errorcluster, "Data"=w388:string, "Command"=w389:string, "RemoteControl.ZMQ out"=w390:refnum<class "RemoteControl.ZMQ.lvclass">, "ID"=w392:string)  [unwired: 5 in]
                n136 = case shown="Default" w389 {
                  selector: w389 -> [w404 _]
                  tunnel: w392 -> [w406 _]
                  tunnel: w391 -> [w409 w419]
                  tunnel: [w409 w419] -> w395
                  tunnel: w390 -> [w405 w415]
                  tunnel: w388 -> [w407 _]
                  tunnel: [enum16{"waiting", "processing"}."processing" ("state") w418] -> w397
                  tunnel: enum16{"waiting", "processing"}."waiting" ("state") -> [_ w418]
                  tunnel: ["RC: Send Message to Owner" ""] -> w396
                  tunnel: [5000 w417] -> w394
                  tunnel: w393 -> [_ w417]
                  tunnel: [w403 T4 {"Command"="", "Data"=variant(string ""), "ID"=""} ("Message out")] -> w381
                  tunnel: [w405 w415] -> w380
                  frame Default {
                    n137 = Bundle By Name(cluster=T4 {"Command"="", "Data"=variant(string ""), "ID"=""} ("Message from Remote"), "Command"=w404, "Data"=w407, "ID"=w406) -> (w403:T4)
                    n138 = call <userlib>:"Format Message String.vi"("ID"=w406, "Data"=w407, "Command"=w404) -> ("Message"=→"Message In":string)  [unwired: 8 in]
                  }
                  frame "" {
                    # "Messages coming from TCP need to have command"
                  }
                }
                n139 = Bundle By Name(cluster=w387, "to"=w394, "state"=w397, "SelfRef"=w380, "Message (in)"=w381) -> (w399:T6)
                n140 = call <vilib>:"Add State(s) to Queue__jki_lib_state_machine.vi"("State(s) in Front (\"\")"=w396, "State(s) in (\"\")"=w402) -> ("States Out"=w401:string)  [unwired: 13 in]
              }
              frame "RC: Write Message" {
                # "After the loop completes\nempty the out queue"
                # "This loop will run # times equal to messages in the out queue"
                # "send Message over, eg. TCP"
                n141 = Unbundle By Name(w430) -> ("SelfRef"=w433:refnum<class "RemoteControl.ZMQ.lvclass">, "Message (out)"=w420:T4)
                n142 = Unbundle By Name(w420) -> ("Command"=w421:string, "Data"=w422:variant, "ID"=w423:string)
                n143 = while {
                  tunnel: w432 -> [w438]
                  tunnel: [w438] -> w424
                  stop <- "delay response" continue-if-true
                }
                n144 = call-dynamic "Send Message.vi"("ID"=w423, "error in (no error)"=w424, "Data"=w422, "Command"=w421, "RemoteControl.ZMQ in"=w433) -> ("error out"=w431:errorcluster, "RemoteControl.ZMQ out"=w425:refnum<class "RemoteControl.ZMQ.lvclass">)  [unwired: 5 in]
                n145 = Bundle By Name(cluster=w430, "Message (out)"=T4 {"Command"="", "Data"=variant, "ID"=""} ("Messages (out)"), "state"=enum16{"waiting", "processing"}."waiting", "to"=5, "SelfRef"=w425) -> (w429:T6)
                n146 = call <vilib>:"Add State(s) to Queue__jki_lib_state_machine.vi"("State(s) in (\"\")"=w436) -> ("States Out"=w435:string)  [unwired: 14 in]
              }
              frame "RC: Close Connection" {
                # "Closes open server connections"
                # "call this on error 66, etc (when connection\ndrops). check these in error handler"
                n147 = Unbundle By Name(w443) -> ("SelfRef"=w444:refnum<class "RemoteControl.ZMQ.lvclass">)
                n148 = call-dynamic "Close Connection.vi"("error in (no error)"=w440, "RemoteControl.ZMQ in"=w444) -> ("error out"=w439:errorcluster, "RemoteControl.ZMQ out"=w441:refnum<class "RemoteControl.ZMQ.lvclass">)  [unwired: 8 in]
                n149 = Bundle By Name(cluster=w443, "SelfRef"=w441) -> (w442:T6)
                n150 = call <vilib>:"Add State(s) to Queue__jki_lib_state_machine.vi"("State(s) in (\"\")"=w447) -> ("States Out"=w446:string)  [unwired: 14 in]
              }
              frame "RC: Open Server Connection" {
                n151 = Unbundle By Name(w456) -> ("SelfRef"=w454:refnum<class "RemoteControl.ZMQ.lvclass">)
                n152 = call-dynamic "Read address.vi"("error in (no error)"=w449, "RemoteControl in"=w454) -> ("error out"=w450:errorcluster, "address"=w455:string, "RemoteControl out"=w453:refnum<class "RemoteControl.ZMQ.lvclass">)  [unwired: 7 in]
                n153 = call-dynamic "Read Port.vi"("error in (no error)"=w450, "RemoteControl in"=w453) -> ("error out"=w448:errorcluster, "Port"=w451:u16, "RemoteControl out"=w452:refnum<class "RemoteControl.ZMQ.lvclass">)  [unwired: 7 in]
                n154 = call-dynamic "Open Server Connection.vi"("error in (no error)"=w448, "Port"=w451, "address"=w455, "RemoteControl.ZMQ in"=w452) -> ("error out"=w459:errorcluster, "RemoteControl.ZMQ out"=w458:refnum<class "RemoteControl.ZMQ.lvclass">)  [unwired: 6 in]
                n155 = Bundle By Name(cluster=w456, "SelfRef"=w458) -> (w457:T6)
                n156 = call <vilib>:"Add State(s) to Queue__jki_lib_state_machine.vi"("State(s) in (\"\")"=w462) -> ("States Out"=w461:string)  [unwired: 14 in]
              }
            }
          }
        }
        frame Error {
        }
      }
      n157 = call-parent "Process_donotrun.vi"("error in (no error)"=w8, "RemoteControl"=w7) -> ("error out"=w5:errorcluster, "RemoteControl out"=w6:refnum<class "RemoteControl.ZMQ.lvclass">)  [unwired: 8 in]
    }
    frame Enabled {
      n158 = disable-structure shown="Disabled" {
        frame Disabled {
          # "Ignore termination error"
          # "It is VERY important we close the context and NOT the socket here, as the socket will be currently IN USE by the blocking receive call most of the time. Destroying something in use causes instability and may crash LabVIEW."
          # "In this case we use the fully blocking receive call. If it returns we know we got something.\nPressing the stop button triggers the event structure which terminates the context, producing an error in the receive loop, which stops and then closes the socket it.\nThis is the preferred implementation, as described in the guide"
          # "LAZY PIRATE PATTERN: Server-side (blocking version)"
          n159 = call <vilib>:"zmq_ctx_create.vi"() -> ("context out"=w470:refnum<class "zmq_context.lvclass">)  [unwired: 4 in, 1 out]
          n160 = call <vilib>:"zmq_socket.vi"("socket type"=socket_type."ZMQ_REP", "context in"=w470) -> ("socket out"=w471:refnum<class "zmq_socket.lvclass">, "context out"=w472:refnum<class "zmq_context.lvclass">)  [unwired: 3 in, 1 out]
          n161 = call <vilib>:"zmq_bind.vi"("endpoint"="endpoint", "socket in"=w471) -> ("socket out"=w467:refnum<class "zmq_socket.lvclass">)  [unwired: 2 in, 1 out]
          n162 = event shown="[0] \"stop?\": Value Change" {
            selector: _ -> [_]
            dyn-events: _ -> [_]
            timeout: _ -> [_]
            tunnel: w472 -> [w476]
            event "stop?": Value Change {
              n163 = event-data() -> ()  [unwired: 1 in, 1 out]
              n164 = call <vilib>:"zmq_ctx_destroy.vi"("context in"=w476) -> ()  [unwired: 4 in, 1 out]
            }
          }
          n165 = while {
            shift-right: [w483] -> w469
            shift-left: w467 -> [w488]
            tunnel: [w480] -> w474
            i -> [w482]
            stop <- w480 stop-if-true
            n166 = call <vilib>:"zmq_recv_multi.vi"("socket in"=w488) -> ("error out"=w481:errorcluster, "parts"=w486:string[], "socket out"=w487:refnum<class "zmq_socket.lvclass">)  [unwired: 2 in]
            n167 = Index Array(array=w486) -> (element=w479:string)  [unwired: 1 in]
            n168 = Decimal String To Number(string=w479) -> (number=w485:i32)  [unwired: 2 in, 1 out]
            n169 = Square(x=w485) -> (x^2=w484:i32)
            n170 = Number To Decimal String(number=w484) -> (decimal integer string=w478:string)  [unwired: 1 in]
            n171 = Build Array(w479, w478) -> (w477:string[])
            n172 = call <vilib>:"zmq_send_multi.vi"("error in"=w481, "parts"=w477, "socket in"=w487) -> ("error out"=w480:errorcluster, "socket out"=w483:refnum<class "zmq_socket.lvclass">)  [unwired: 1 in]
            "loop" <- w482
          }
          n173 = call <vilib>:"zmq_check_term.vi"("error in"=w474) -> ("error out"=w475:errorcluster)  [unwired: 1 in, 1 out]
          n174 = call <vilib>:"zmq_close.vi"("error in"=w475, "socket"=w469) -> ("error out"=w473:errorcluster)  [unwired: 3 in]
          n175 = call <vilib>:"Clear Errors.vi"("error in (no error)"=w473) -> ()  [unwired: 5 in, 2 out]
        }
        frame Enabled {
        }
      }
    }
  }
  "RemoteControl.ZMQ out" <- w2
  "error out" <- w1
